vi "radial_0707V1.vi"() -> ()   [LabVIEW 2013]
uses:
  <vilib>/Utility/error.llb/DialogType.ctl
  <vilib>/DAQmx/read.llb/DAQmx Read (Analog 2D DBL NChan NSamp).vi
  <vilib>/DAQmx/read.llb/DAQmx Read (Digital 1D Wfm NChan NSamp).vi
  <vilib>/DAQmx/create/channels.llb/DAQmx Create Channel (DI-Digital Input).vi
  <vilib>/DAQmx/configure/timing.llb/DAQmx Timing (Sample Clock).vi
  <vilib>/Utility/file.llb/Read From Spreadsheet File (DBL).vi
  <vilib>/gmath/interp.llb/Interpolate 2D Scattered (2D).vi
  <vilib>/Math Plots/3D Math Plots/3D Scatter/3D Scatter Datatype/Public/Plot Helper (Vector).vi
  <vilib>/Waveform/DTblOps.llb/DTbl Digital to Boolean Array.vi
  <vilib>/DAQmx/miscellaneous.llb/DAQmx Fill In Error Info.vi
  <vilib>/DAQmx/create/channels.llb/DAQmx Create Channel (AI-Voltage-Basic).vi
  <resource>/objmgr/daqmx.rc
  <vilib>/Math Plots/3D Math Plots/3D Scatter/3D Scatter Datatype/3D Scatter Datatype.lvclass
  <vilib>/gmath/NI_AAL_Interpolation.lvlib
panel:
  out "XYZ Data":cluster{"X":dbl[], "Y":dbl[], "Z":dbl[]}
  out "Finish moving":bool
  in  "name or relative path":string="data\\0629n1_80V"
  out "K":dbl
  out "Speed":dbl
  out "B-EMF":dbl[](graph)=[0.07481589133166745, 0.07511337105786742, 0.0741529055838003, 0.07537265906376046, 0.07508825632115766, 0.07557435638030187, 0.0743975577603694, 0.07492228255252237, 0.07463056189525759, 0.0758438201846894, 0.07482290613743812, 0.07511679185821236, 0.07415273237871953, 0.07537876454285714, 0.07509791250440986, 0.07558596112071256, 0.0743927080181082, 0.07491881845090724, 0.07463770660483883, 0.07585304335523971, 0.07481316335164553, 0.07513961162760209, 0.07414004510655407, 0.0753934869747215, 0.07509271635198714, 0.07559592041285612, 0.07439296782572931, 0.07493276145990817, 0.07463588795149087, 0.07587720546400528, 0.07480203492520691, 0.07514974412482635, 0.07413324680713437, 0.07542358135750299, 0.07508440250811083, 0.07560570649991886, 0.07438603962249907, 0.07495536472294693, 0.07461891385357669, 0.07588144898848384, 0.07480381027728465, 0.07516195508301972, 0.07413138485251623, 0.07541942443556485, 0.07507565565153261, 0.07562294040545418, 0.07437421837573739, 0.07496484770111837, 0.07462229135265147, 0.07589993863085463, 0.07480216482901747, 0.07518568417908342, 0.07412164206672368, 0.07543691814872129, 0.07506110642474902, 0.07564398482276614, 0.07437668654813819, 0.07498160529268162, 0.07461267847066942, 0.0759097247179174, 0.07477362929196277, 0.07519404132422994, 0.07411445405587225, 0.07546108025748688, 0.07506634587844192, 0.07565281828188475, 0.07436131459722098, 0.07499658753216708, 0.07460471103695462, 0.07593150525682257, 0.0747739324008541, 0.07521118862722488, 0.07411661911938174, 0.075469350800093, 0.07505032440847191, 0.07567741340335221, 0.07435451629780128, 0.07502092284601342, 0.07459782613499454, 0.0759478731369541, 0.07476483913411439, 0.07523058759626963, 0.07409336633729012, 0.07548000291255955, 0.07504733662082885, 0.07569139971362333, 0.07435061918348428, 0.0750335235156385, 0.0745818912675649, 0.07596948047077853, 0.07476141833376944, 0.07525267124406612, 0.07408821348613759, 0.07550827864199311, 0.07503378332325962, 0.07571058217631717, 0.07433632976432183, 0.07505898466250974, 0.0745710659500176, 0.07598351008231984, 0.07475838724485617, 0.07526722047084973, 0.07407912021939786, 0.07552399700307182, 0.07501602980248206, 0.07573383495840878, 0.0743232094794545, 0.07508344988016666, 0.07455508778131775, 0.07600464110217219, 0.07473353231576757, 0.07529501988631122, 0.07406253583291537, 0.0755460806508683, 0.07500832217638835, 0.07575197819061805, 0.07430298778627613, 0.07510068378570196, 0.0745526629101872, 0.07604226990596659, 0.0747173376407168, 0.07531303321470993, 0.07405010836837107, 0.07557439968157206, 0.074991304777204, 0.07578306850261392, 0.07429489044875075, 0.0751250624008185, 0.07452858740396197, 0.07605456746670036, 0.07470581950284645, 0.0753423914758982, 0.07402646587484775, 0.07559358214426588, 0.07497147279545732, 0.07580671099613724, 0.07426800035996324, 0.07516173857666877, 0.07450693676886735, 0.07607426954463645, 0.07468577101474887, 0.07537097031422309, 0.07399957578606026, 0.07563593078651094, 0.07496328885539158, 0.0758321721430085, 0.07424877459599921, 0.07519157315182916, 0.07447896414832511, 0.07611419331575092, 0.07466234502757649, 0.07539301066074941, 0.07397181967186896, 0.07566411991340413, 0.07492154643092916, 0.07586607703756665, 0.0742194596360811, 0.07522162423334047, 0.07445055851508102, 0.07615680176561711, 0.07463056189525759, 0.07543172199629856, 0.07394415016021806, 0.07570560253024541, 0.0748928376887937, 0.07590998452553853, 0.07418278346023084, 0.07526743697720066, 0.07441184717953182, 0.07620157527899274, 0.07459211036732954, 0.0754861949941966, 0.07390513571577755, 0.075761114758628, 0.07485213449481584, 0.07596172954341465, 0.07414134414465974, 0.07530259760859431, 0.0]
  in  "Tab Control":enum32{"Setting"}(tab)
  in  "move":bool caption="OK Button 3"
  in  "Auto Run":bool caption="OK Button 3"
  out "Finish Save Data":bool
  in  "Save Data":bool caption="stop"
  out "Waveform Graph":dbl[][](graph)
  in  "Optical scale":tag="PXI1Slot5/port0/line0:2"
  in  "Rate":dbl=100000.0 caption="Input Rate" format="%0.2f"
  out "Position Check?":bool
  out "Position":dbl
  out "SampClk.Rate":dbl
  out "Waveform Chart":dbl(graph)
  in  "Stop to all":bool caption="stop"
  in  "Input Channel":tag="PXI1Slot5/ai6" caption="A.I.Physical Channel"
  out "Speed(rad/s)":dbl[](graph)
  in  "Storage Times":dbl=10.0 format="%#_13g"
  in  "Maximum":dbl=1.0 caption="Maximum Value" format="%0.2f"
  in  "Minimum":dbl=-1.0 caption="Minimum Value" format="%0.2f"
  in  "Auto Array":dbl[](array[numeric])=[0.0, -2.0, -4.0, -6.0, -10.0, -15.0, -20.0, -25.0]
  in  "Stop":bool caption="OK Button 3"
  in  "y":dbl=10.0 format="%#_13g"
  # "Move"
  # "Air Gap Distance"
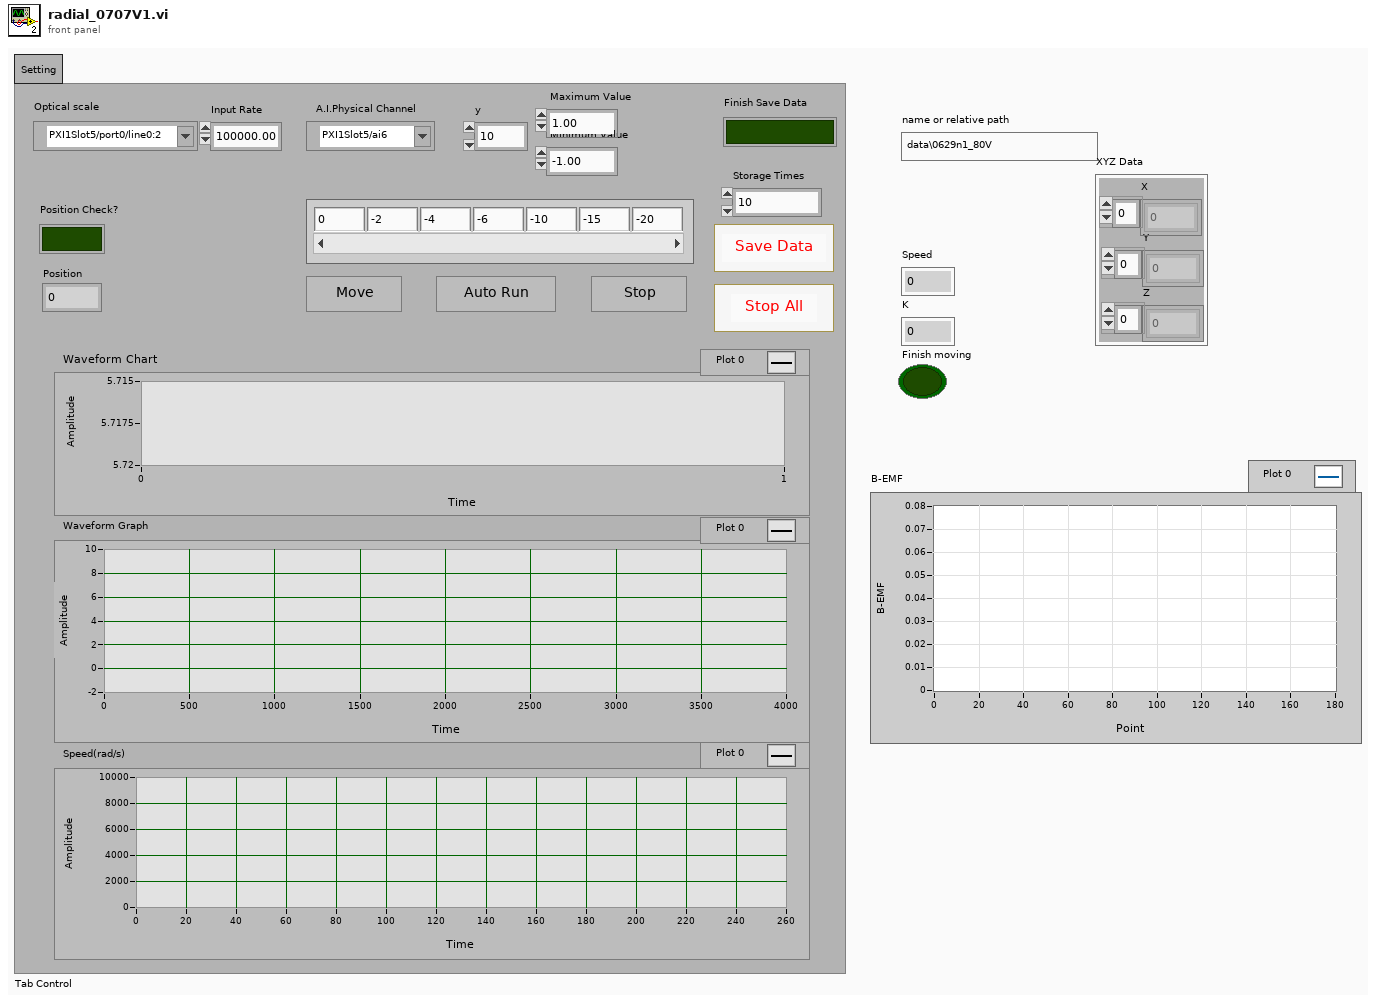
[diagram p1: front panel]
types:
  T1 = typedef "DialogType.ctl" = u16
  T2 = cluster{"Speed":dbl, "Torque":dbl, "K":dbl, "Air gap distance ":dbl, "Torque_O":dbl}
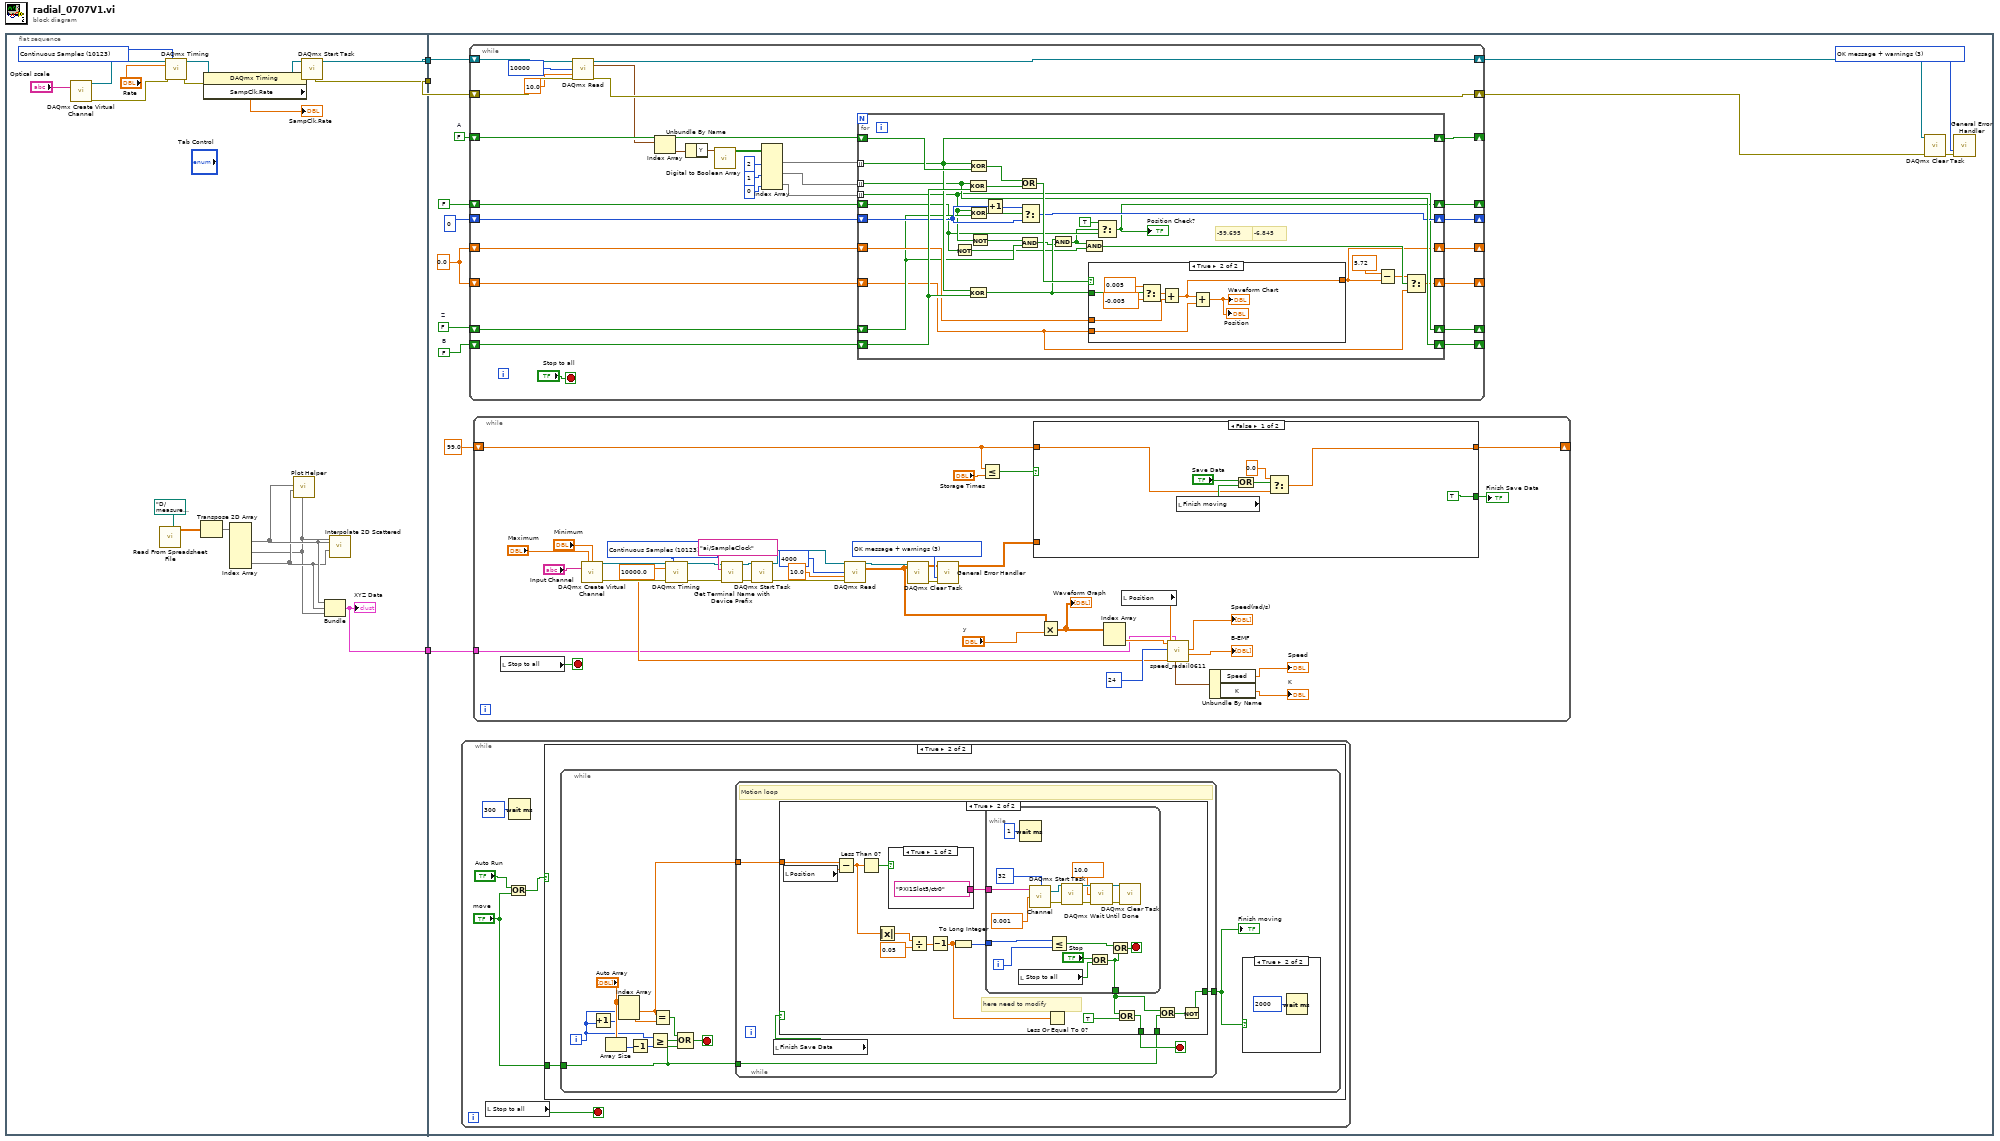
[diagram p0: block diagram]
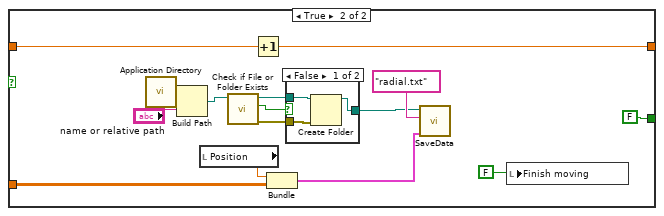
[diagram p2: hidden frame]
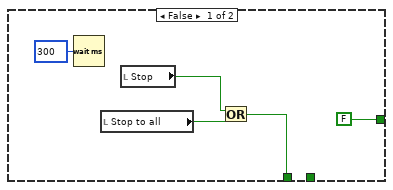
[diagram p6: hidden frame]
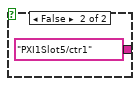
[diagram p7: hidden frame]
diagram:
  n1 = flat-sequence {
    tunnel: [w13] -> w3
    tunnel: [w12] -> w2
    tunnel: [w4] -> w1
    tunnel: w3 -> [w29]
    tunnel: w2 -> [w28]
    tunnel: w1 -> [w23]
    frame #0 {
      w16 = 10123 items=["Finite Samples"=10178, "Continuous Samples"=10123] ("sample mode")
      n2 = call-poly <vilib>:"DAQmx Create Virtual Channel.vi"("lines"="Optical scale") -> ("task out"=w15:refnum<k21>, "error out"=w14:errorcluster)  [unwired: 13 in]
      n3 = call-poly <vilib>:"Read From Spreadsheet File.vi"("file path (dialog if empty)"=path "D:/measurement/coupling/raidl_coupling/TNposition.txt") -> ("all rows"=w9:dbl[][])  [unwired: 6 in, 4 out]
      n4 = call-poly <vilib>:"DAQmx Timing.vi"("task/channels in"=w15, "sample mode"=w16, "rate"="Rate", "error in"=w14) -> ("task out"=w18:refnum<k21>, "error out"=w17:errorcluster)  [unwired: 10 in]
      n5 = Transpose 2D Array(2D array=w9) -> (transposed array=w8:dbl[][])
      n6 = property class="DAQmx Timing"(reference=w18, error in=w17) -> (reference out=w19:refnum<k21>, error out=w20:errorcluster, "SampClk.Rate"=→"SampClk.Rate":dbl)
      n7 = Index Array(array=w8) -> (element #1=w7:dbl[], element #2=w5:dbl[], element #3=w6:dbl[])  [unwired: 6 in]
      n8 = call-poly <vilib>:"Plot Helper.vi"("z vector"=w5, "y vector"=w6, "x vector"=w7) -> ()  [unwired: 3 in, 6 out]
      n9 = call <vilib>:"DAQmx Start Task.vi"("task/channels in"=w19, "error in"=w20) -> ("task out"=w13:refnum<k21>, "error out"=w12:errorcluster)  [unwired: 12 in]
      n10 = Bundle(w7, w6, w5) -> (w4:cluster{dbl[], dbl[], dbl[]})  [unwired: 1 in]
      "XYZ Data" <- w4
      n11 = call-poly <vilib>:"Interpolate 2D Scattered.vi"("Y"=w6, "X"=w7, "Z"=w5) -> ()  [unwired: 7 in, 2 out]
    }
    frame #1 {
      w24 = FALSE  # B
      w27 = FALSE  # A
      w25 = 0.0
      w32 = FALSE  # Z
      w35 = T1 3 items=["no dialog", "OK message", "continue or stop message", "OK message + warnings", "continue/stop + warnings"] ("type of dialog (OK msg:1)")
      n12 = while {
        stop <- w103 stop-if-true
        n13 = local read "Stop to all"() -> (w103:bool)
        n14 = Or(x="Auto Run", y="move") -> (x .or. y?=w101:bool)
        n15 = Wait (ms)(milliseconds to wait=u32 300) -> ()  [unwired: 1 out]
        n16 = case shown="True" w101 {
          tunnel: "move" -> [_ w105]
          frame False {
          }
          frame True {
            n17 = while {
              tunnel: w105 -> [w107]
              i -> [w116]
              stop <- w106 stop-if-true
              n18 = Increment(x=w116) -> (x+1=w112:i32)
              n19 = Array Size(array="Auto Array") -> (size(s)=w108:i32)
              n20 = Index Array(array="Auto Array", index #1=w116, index #2=w112) -> (element #1=w115:dbl, element #2=w111:dbl)
              n21 = Decrement(x=w108) -> (x-1=w109:i32)
              n22 = Greater Or Equal?(x=w116, y=w109) -> (x >= y?=w113:bool)
              n23 = Equal?(x=w115, y=w111) -> (x = y?=w114:bool)
              n24 = Compound Arithmetic op=OR(w114, w113, w107) -> (w106:bool)
              n25 = while {
                tunnel: w115 -> [w123]
                tunnel: [w121] -> w110
                tunnel: w107 -> [w119]
                stop <- w122 stop-if-true
                # "Motion loop"
                n26 = local read "Finish Save Data"() -> (w120:bool)
                n27 = case shown="True" w120 {
                  tunnel: w123 -> [_ w139]
                  tunnel: [w125 w134] -> w122
                  tunnel: [FALSE w133] -> w121
                  tunnel: w119 -> [_ w131]
                  frame False {
                    n28 = Wait (ms)(milliseconds to wait=u32 300) -> ()  [unwired: 1 out]
                    n29 = local read "Stop to all"() -> (w127:bool)
                    n30 = local read "Stop"() -> (w126:bool)
                    n31 = Or(x=w126, y=w127) -> (x .or. y?=w125:bool)
                  }
                  frame True {
                    # "here need to modify"
                    n32 = local read "Position"() -> (w140:dbl)
                    n33 = Subtract(x=w139, y=w140) -> (x-y=w137:dbl)
                    n34 = Less Than 0?(x=w137) -> (x < 0?=w136:bool)
                    n35 = Absolute Value(x=w137) -> (abs(x)=w138:dbl)
                    n36 = case shown="True" w136 {
                      tunnel: ["PXI1Slot5/ctr0" ("counter") "PXI1Slot5/ctr1" ("counter")] -> w141
                      frame True {
                      }
                      frame False {
                      }
                    }
                    n37 = Divide(x=w138, y=0.05) -> (x/y=w143:dbl)
                    n38 = Decrement(x=w143) -> (x-1=w135:dbl)
                    n39 = To Long Integer(number=w135) -> (32bit integer=w142:i32)
                    n40 = while {
                      tunnel: w142 -> [w157]
                      tunnel: w141 -> [w155]
                      tunnel: [w148] -> w130
                      i -> [w154]
                      stop <- w151 stop-if-true
                      n41 = local read "Stop to all"() -> (w149:bool)
                      n42 = Wait (ms)(milliseconds to wait=u32 1) -> ()  [unwired: 1 out]
                      n43 = call "Channel.vi"("number of samples"=32, "High & Low time"=0.001, "counter"=w155) -> ("error out"=w163:errorcluster, "task out"=w164:refnum<k21>)  [unwired: 1 in]
                      n44 = Less Or Equal?(x=w157, y=w154) -> (x <= y?=w152:bool)
                      n45 = call <vilib>:"DAQmx Start Task.vi"("task/channels in"=w164, "error in"=w163) -> ("task out"=w160:refnum<k21>, "error out"=w159:errorcluster)  [unwired: 12 in]
                      n46 = Or(x="Stop", y=w149) -> (x .or. y?=w148:bool)
                      n47 = call <vilib>:"DAQmx Wait Until Done.vi"("task/channels in"=w160, "timeout (sec)"=10.0 ("timeout (s)"), "error in"=w159) -> ("task out"=w162:refnum<k21>, "error out"=w161:errorcluster)  [unwired: 11 in]
                      n48 = Or(x=w152, y=w148) -> (x .or. y?=w151:bool)
                      n49 = call <vilib>:"DAQmx Clear Task.vi"("task in"=w162, "error in"=w161) -> ()  [unwired: 13 in, 1 out]
                    }
                    n50 = Less Or Equal To 0?(x=w135) -> ()  [unwired: 1 out]
                    n51 = Or(x=w130, y=TRUE) -> (x .or. y?=w134:bool)
                    n52 = Or(x=w130, y=w131) -> (x .or. y?=w129:bool)
                    n53 = Not(x=w129) -> (.not. x?=w133:bool)
                  }
                }
              }
              "Finish moving" <- w110
              n54 = case shown="True" w110 {
                frame False {
                }
                frame True {
                  n55 = Wait (ms)(milliseconds to wait=u32 2000) -> ()  [unwired: 1 out]
                }
              }
            }
          }
        }
      }
      n56 = while {
        shift-right: [w180] -> w34
        shift-left: w29 -> [w181]
        shift-right: [w195] -> w33
        shift-left: w28 -> [w194]
        shift-right: [w187] -> _
        shift-left: w27 -> [w185]
        shift-right: [w186] -> _
        shift-left: w24 -> [w184]
        shift-right: [w183] -> _
        shift-left: w25 -> [w182]
        shift-right: [w175] -> _
        shift-left: w32 -> [w177]
        shift-right: [w173] -> _
        shift-left: 0 -> [w174]
        shift-right: [w172] -> _
        shift-left: FALSE ("X4?") -> [w167]
        shift-right: [w170] -> _
        shift-left: w25 -> [w171]
        stop <- "Stop to all" stop-if-true
        n57 = call-poly <vilib>:"DAQmx Read.vi"("task/channels in"=w181, "number of samples per channel"=10000, "timeout"=10.0, "error in"=w194) -> ("task out"=w180:refnum<k21>, "data"=w165:digitalwaveform[], "error out"=w195:errorcluster)  [unwired: 9 in]
        n58 = Index Array(array=w165) -> (element=w191:digitalwaveform)  [unwired: 1 in]
        n59 = Unbundle By Name(w191) -> ("Y"=w192:digitaldata)
        n60 = call-poly <vilib>:"Digital to Boolean Array.vi"("digital data"=w192) -> ("boolean array"=w190:bool[][])  [unwired: 9 in, 1 out]
        n61 = Index Array(array=w190, index (col) #1=2 ("disabled index (col)"), index (col) #2=1 ("disabled index (col)"), index (col) #3=0 ("index (col)")) -> (element #1=w166:bool[], element #2=w179:bool[], element #3=w176:bool[])  [unwired: 3 in]
        n62 = for {
          tunnel: w166 -> [w221] mode=indexing
          tunnel: w179 -> [w218] mode=indexing
          shift-right: [w221] -> w187
          shift-left: w185 -> [w223]
          shift-right: [w218] -> w186
          shift-left: w184 -> [w222]
          shift-right: [w197] -> w183
          shift-left: w182 -> [w219]
          shift-right: [w208] -> w175
          shift-left: w177 -> [w210]
          tunnel: w176 -> [w208] mode=indexing
          shift-right: [w214] -> w173
          shift-left: w174 -> [w215]
          shift-right: [w196] -> w172
          shift-left: w167 -> [w205]
          shift-right: [w201] -> w170
          shift-left: w171 -> [w200]
          # "-6.845"
          # "-59.695"
          n63 = Not(x=w205) -> (.not. x?=w204:bool)
          n64 = Exclusive Or(1:w222, 2:w218) -> (0:w212:bool)
          n65 = Exclusive Or(1:w222, 2:w221) -> (0:w211:bool)
          n66 = Exclusive Or(1:w223, 2:w221) -> (0:w213:bool)
          n67 = Exclusive Or(1:w210, 2:w208) -> (0:w217:bool)
          n68 = Not(x=w208) -> (.not. x?=w209:bool)
          n69 = Increment(x=w215) -> (x+1=w216:i32)
          n70 = Or(x=w213, y=w212) -> (x .or. y?=w220:bool)
          n71 = And(x=w209, y=w210) -> (x .and. y?=w207:bool)
          n72 = Select(t=w216, s=w217, f=w215) -> (s? t:f=w214:i32)
          n73 = And(x=w211, y=w207) -> (x .and. y?=w203:bool)
          n74 = And(x=w203, y=w204) -> (x .and. y?=w202:bool)
          n75 = case shown="True" w220 {
            tunnel: [w224 w227] -> w197
            tunnel: w219 -> [w224 w230]
            tunnel: w211 -> [_ w231]
            tunnel: w200 -> [_ w225]
            frame False {
            }
            frame True {
              n76 = Select(t=0.005, s=w231, f=-0.005 ("t")) -> (s? t:f=w229:dbl)
              n77 = Add(x=w229, y=w230) -> (x+y=w227:dbl)
              n78 = Add(x=w227, y=w225) -> (x+y=→"Waveform Chart" →"Position":dbl)
            }
          }
          n79 = Select(t=TRUE, s=w203, f=w205) -> (s? t:f=w196:bool)
          "Position Check?" <- w196
          n80 = Subtract(x=5.72 ("t"), y=w197) -> (x-y=w199:dbl)
          n81 = Select(t=w199, s=w202, f=w200) -> (s? t:f=w201:dbl)
        }
      }
      n82 = while {
        shift-right: [w55] -> _
        shift-left: 99.0 -> [w54]
        tunnel: w23 -> [w37]
        stop <- w40 stop-if-true
        w60 = T1 3 items=["no dialog", "OK message", "continue or stop message", "OK message + warnings", "continue/stop + warnings"] ("type of dialog (OK msg:1)")
        w73 = 10123 items=["Finite Samples"=10178, "Continuous Samples"=10123] ("sample mode")
        w47 = 10000.0 ("rate")
        n83 = local read "Stop to all"() -> (w40:bool)
        n84 = call-poly <vilib>:"DAQmx Create Virtual Channel.vi"("maximum value"="Maximum", "minimum value"="Minimum", "physical channels"="Input Channel") -> ("task out"=w69:refnum<k21>, "error out"=w68:errorcluster)  [unwired: 11 in]
        n85 = call-poly <vilib>:"DAQmx Timing.vi"("task/channels in"=w69, "sample mode"=w73, "rate"=w47, "error in"=w68) -> ("task out"=w71:refnum<k21>, "error out"=w70:errorcluster)  [unwired: 10 in]
        n86 = call "Get Terminal Name with Device Prefix.vi"("error in (no error)"=w70, "Local Terminal Name"="ai/SampleClock", "task/channels in"=w71) -> ("error out"=w62:errorcluster, "task out"=w63:refnum<k21>)  [unwired: 6 in, 1 out]
        n87 = call <vilib>:"DAQmx Start Task.vi"("task/channels in"=w63, "error in"=w62) -> ("task out"=w65:refnum<k21>, "error out"=w64:errorcluster)  [unwired: 12 in]
        n88 = call-poly <vilib>:"DAQmx Read.vi"("task/channels in"=w65, "number of samples per channel"=4000, "timeout"=10.0, "error in"=w64) -> ("task out"=w59:refnum<k21>, "data"=w52:dbl[][])  [unwired: 9 in, 1 out]
        n89 = call <vilib>:"DAQmx Clear Task.vi"("task in"=w59) -> ("error out"=w61:errorcluster)  [unwired: 14 in]
        n90 = call <vilib>:"General Error Handler.vi"("type of dialog (OK msg:1)"=w60, "error in (no error)"=w61) -> ()  [unwired: 9 in, 5 out]
        n91 = Less Or Equal?(x=w54, y="Storage Times") -> (x <= y?=w53:bool)
        n92 = case shown="False" w53 {
          tunnel: w52 -> [_ w95]
          tunnel: [w74 w92] -> w55
          tunnel: w54 -> [w75 w91]
          tunnel: [TRUE ("Boolean") FALSE ("Boolean")] -> w44
          frame False {
            n93 = local read "Finish moving"() -> (w78:bool)
            n94 = Or(x="Save Data", y=w78) -> (x .or. y?=w77:bool)
            n95 = Select(t=0.0, s=w77, f=w75) -> (s? t:f=w74:dbl)
          }
          frame True {
            n96 = call <vilib>:"Application Directory.vi"() -> ("Application Directory"=w83:path)
            n97 = Build Path(base path=w83, name or relative path="name or relative path") -> (appended path=w84:path)
            n98 = local read "Position"() -> (w94:dbl)
            n99 = call <vilib>:"Check if File or Folder Exists.vi"("path"=w84) -> ("error out"=w87:errorcluster, "file or folder exists?"=w85:bool, "dup path"=w86:path)  [unwired: 8 in]
            n100 = Increment(x=w91) -> (x+1=w92:dbl)
            n101 = Bundle("Position"=w94, "data"=w95) -> (w93:cluster{"Position":dbl, "data":dbl[][]})  [unwired: 1 in]
            n102 = case shown="False" w85 {
              tunnel: w86 -> [w98 w99]
              tunnel: w87 -> [w97 _]
              tunnel: [w96 w99] -> w81
              frame False {
                n103 = Create Folder(path (use dialog)=w98, error in=w97) -> (created path=w96:path)  [unwired: 1 in, 2 out]
              }
              frame True {
              }
            }
            n104 = call "SaveData.vi"("output cluster"=w93, "File name"="radial.txt", "File path"=w81) -> ()  [unwired: 2 in]
            n105 = local write "Finish moving"(FALSE ("Boolean")) -> ()
          }
        }
        "Finish Save Data" <- w44
        n106 = Multiply(x=w52, y="y") -> (x*y=w51:dbl[][])
        "Waveform Graph" <- w51
        n107 = Index Array(array=w51) -> (element=w50:dbl[])  [unwired: 2 in]
        n108 = local read "Position"() -> (w49:dbl)
        n109 = call "speed_radail0611.vi"("XYZ Data"=w37, "rate"=w47, "Optical"=w49, "Pole Pair"=24, "Voltage"=w50) -> ("B-EMF"=→"B-EMF":dbl[], "Speed(rad/s)"=→"Speed(rad/s)":dbl[], "output Data"=w43:T2)  [unwired: 1 in, 2 out]
        n110 = Unbundle By Name(w43) -> ("Speed"=→"Speed":dbl, "K"=→"K":dbl)
      }
      n111 = call <vilib>:"DAQmx Clear Task.vi"("task in"=w34, "error in"=w33) -> ("error out"=w36:errorcluster)  [unwired: 13 in]
      n112 = call <vilib>:"General Error Handler.vi"("type of dialog (OK msg:1)"=w35, "error in (no error)"=w36) -> ()  [unwired: 9 in, 5 out]
    }
  }
